vi "Write.vi"(4 "Buffer Capacity (Bytes)":i32=102400, 5 "Maximum File Size (Bytes)":i64, 6 "File Extension":string="csv", 7 "Maximum File Count":i32, 8 "Error In":errorcluster, 9 "Enable Calendar Tree":bool=TRUE, 10 "Messages":T1[](array[typedef]), 11 "Log In":refnum<file>) -> (0 "Error Out":errorcluster, 3 "Log Out":refnum<file>)   [LabVIEW 2015, in "Logger.lvlib" / "File.lvlib"]
uses:
  File.lvlib
  Public/Controls/Message.ctl
  Public/Controls/Tag.ctl
  Create ISO 8601 File Name.vi
  Write Header.vi
  Create Calendar Folder Tree.vi
  Get Oldest File.vi
  <vilib>/Utility/libraryn.llb/Check if File or Folder Exists.vi
  Logger.lvlib
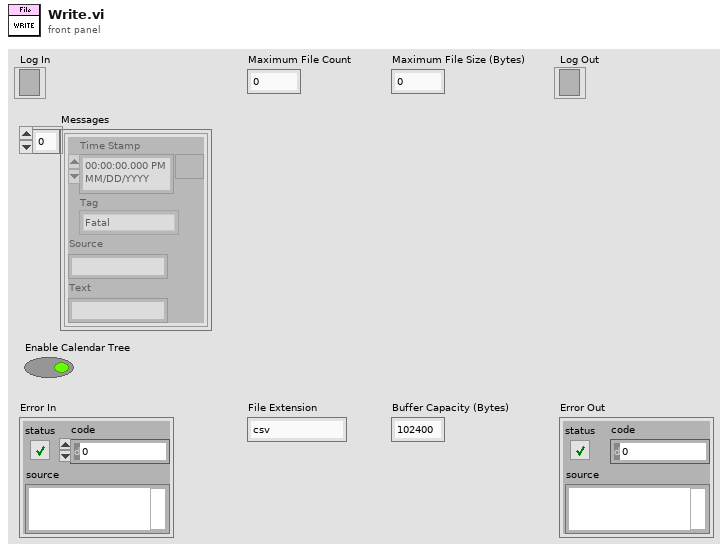
[diagram p1: front panel]
types:
  T1 = typedef "Logger.lvlib/Message.ctl" = cluster{"Time Stamp":timestamp, "Tag":T2, "Source":string, "Text":string}
  T2 = typedef "Logger.lvlib/Tag.ctl" = enum16{"Fatal", "Error", "Warn", "Info", "Debug", "Trace"}
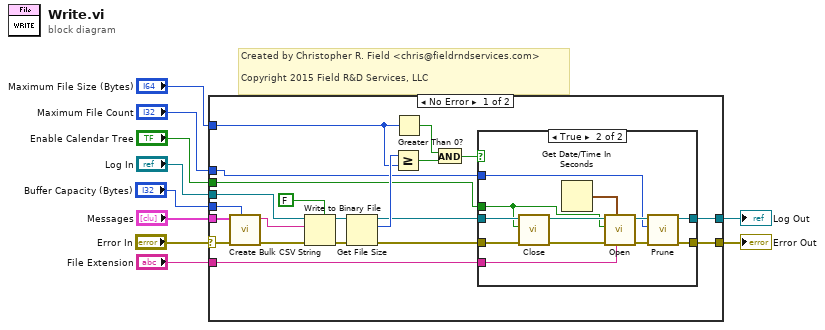
[diagram p0: block diagram]
diagram:
  # "Created by Christopher R. Field <chris@fieldrndservices.com>\n\nCopyright 2015 Field R&D Services, LLC"
  n1 = case shown="No Error" "Error In" {
    selector: "Error In" -> [w15 w46]
    tunnel: "Log In" -> [w31 w47]
    tunnel: "Messages" -> [w14 _]
    tunnel: [w21 w47] -> w7
    tunnel: [w20 w46] -> w6
    tunnel: "Maximum File Size (Bytes)" -> [w22 _]
    tunnel: "Enable Calendar Tree" -> [w19 _]
    tunnel: "Maximum File Count" -> [w18 _]
    tunnel: "File Extension" -> [w17 _]
    tunnel: "Buffer Capacity (Bytes)" -> [w11 _]
    frame No Error {
      n2 = call "Create Bulk CSV String.vi"("Buffer Capacity (Bytes)"=w11, "Error In"=w15, "Messages"=w14) -> ("Error Out"=w12:errorcluster, "Bulk CSV"=w13:string)  [unwired: 7 in]
      n3 = Write to Binary File(file (use dialog)=w31, data=w13, error in=w12, 5:FALSE ("prepend array or string size? (T)")) -> (refnum out=w24:refnum<file>, error out=w23:errorcluster)  [unwired: 2 in, 1 out]
      n4 = Get File Size(file=w24, error in=w23) -> (refnum out=w26:refnum<file>, size (in bytes)=w28:i64, 0:w25:errorcluster)
      n5 = Greater Or Equal?(x=w28, y=w22) -> (x >= y?=w30:bool)
      n6 = Greater Than 0?(x=w22) -> (x > 0?=w29:bool)
      n7 = And(x=w29, y=w30) -> (x .and. y?=w27:bool)
      n8 = case shown="True" w27 {
        tunnel: [w33 w37] -> w21
        tunnel: [w32 w38] -> w20
        tunnel: w26 -> [w33 w44]
        tunnel: w25 -> [w32 w43]
        tunnel: w19 -> [_ w35]
        tunnel: w18 -> [_ w36]
        tunnel: w17 -> [_ w34]
        frame False {
        }
        frame True {
          n9 = call "Close.vi"("Error In"=w43, "Enable Calendar Tree"=w35, "Log In"=w44) -> ("Error Out"=w42:errorcluster, "Base Log Folder"=w41:path)  [unwired: 7 in]
          n10 = Get Date/Time In Seconds() -> (seconds since 1Jan1904=w45:timestamp)
          n11 = call "Open.vi"("File Extension"=w34, "Start Time Stamp"=w45, "Error In"=w42, "Enable Calendar Tree"=w35, "Base Folder"=w41) -> ("Error Out"=w39:errorcluster, "Log Out"=w40:refnum<file>)  [unwired: 5 in]
          n12 = call "Prune.vi"("Error In"=w39, "Maximum File Count"=w36, "File In"=w40) -> ("Error Out"=w38:errorcluster, "File Out"=w37:refnum<file>)  [unwired: 7 in]
        }
      }
    }
    frame Error {
    }
  }
  "Log Out" <- w7
  "Error Out" <- w6
